vi "aotf_do_waveform_multiD.vi"(0 "Actual Sweep Time (µS)":u32, 5 "Sweep Interval (µS)":u32, 7 "Number of Slices":u32, 9 "Left Padding":u32, 11 "Right Padding":u32) -> (8 "Digital Waveform Graph":digitalwaveform(graph))   [LabVIEW 2013]
uses:
  <vilib>/Waveform/DWDTOps.llb/Digital Pattern Generator (Single Value).vi
  <vilib>/Waveform/DWDTOps.llb/DWDT Append Digital Samples.vi
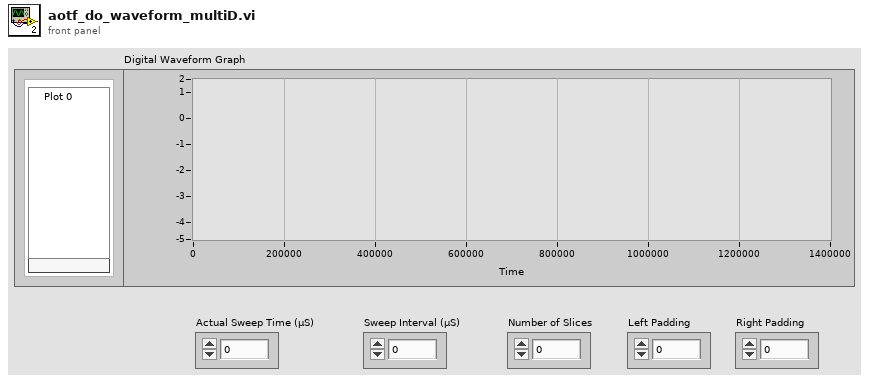
[diagram p1: front panel]
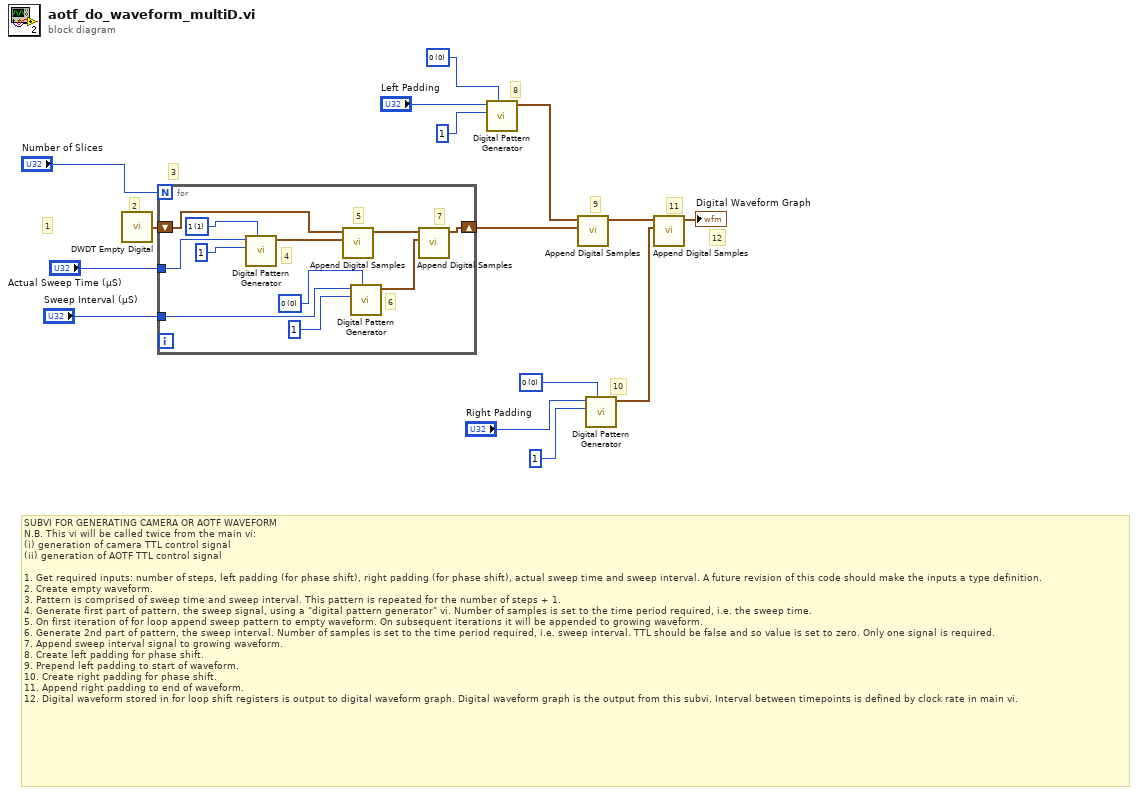
[diagram p0: block diagram]
diagram:
  w7 = u8 0 items=["0", "1", "Z", "L", "H", "X", "T", "V"] ("value")
  w10 = u8 0 items=["0", "1", "Z", "L", "H", "X", "T", "V"] ("value")
  # "12"
  # "11"
  # "10"
  # "9"
  # "8"
  # "3"
  # "2"
  # "1"
  # "SUBVI FOR GENERATING CAMERA OR AOTF WAVEFORM\nN.B. This vi will be called twice from the main vi: \n(i) generation of camera TTL control signal\n(ii) generation of AOTF TTL control signal\n\n1. Get required inputs: number of steps, left padding (for phase shift), right padding (for phase shift), actual sweep time and sweep interval. A future revision of this code should make the inputs a type definition.\n2. Create empty waveform.\n3. Pattern is comprised of sweep time and sweep interval. This pattern is repeated for the number of steps + 1.\n4. Generate first part of pattern, the sweep signal, using a \"digital pattern generator\" vi. Number of samples is set to the time period required, i.e. the sweep time.\n5. On first iteration of for loop append sweep pattern to empty waveform. On subsequent iterations it will be appended to growing waveform.\n6. Generate 2nd part of pattern, the sweep interval. Number of samples is set to the time period required, i.e. sweep interval. TTL should be false and so value is set to zero. Only one signal is required. \n7. Append sweep interval signal to growing waveform.\n8. Create left padding for phase shift.\n9. Prepend left padding to start of waveform.\n10. Create right padding for phase shift.\n11. Append right padding to end of waveform.\n12. Digital waveform stored in for loop shift registers is output to digital waveform graph. Digital waveform graph is the output from this subvi. Interval between timepoints is defined by clock rate in main vi."
  n1 = call <vilib>:"DWDT Empty Digital.vi"() -> ("digital waveform out"=w15:digitalwaveform)  [unwired: 5 in]
  n2 = for {
    N: "Number of Slices" -> [_]
    shift-right: [w16] -> w5
    shift-left: w15 -> [w17]
    tunnel: "Actual Sweep Time (µS)" -> [w20]
    tunnel: "Sweep Interval (µS)" -> [w19]
    w24 = u8 0 items=["0", "1", "Z", "L", "H", "X", "T", "V"] ("value")
    w26 = u8 1 items=["0", "1", "Z", "L", "H", "X", "T", "V"] ("value")
    # "7"
    # "6"
    # "5"
    # "4"
    n3 = call-poly <vilib>:"Digital Pattern Generator.vi"("value"=w26, "number of signals"=u32 1, "number of samples"=w20) -> ("digital waveform"=w22:digitalwaveform)  [unwired: 7 in, 1 out]
    n4 = call-poly <vilib>:"Append Digital Samples.vi"("digital waveform B"=w22, "digital waveform A"=w17) -> ("digital waveform out"=w21:digitalwaveform)  [unwired: 8 in, 1 out]
    n5 = call-poly <vilib>:"Digital Pattern Generator.vi"("value"=w24, "number of signals"=u32 1, "number of samples"=w19) -> ("digital waveform"=w18:digitalwaveform)  [unwired: 7 in, 1 out]
    n6 = call-poly <vilib>:"Append Digital Samples.vi"("digital waveform B"=w18, "digital waveform A"=w21) -> ("digital waveform out"=w16:digitalwaveform)  [unwired: 8 in, 1 out]
  }
  n7 = call-poly <vilib>:"Digital Pattern Generator.vi"("value"=w7, "number of signals"=u32 1, "number of samples"="Left Padding") -> ("digital waveform"=w6:digitalwaveform)  [unwired: 7 in, 1 out]
  n8 = call-poly <vilib>:"Append Digital Samples.vi"("digital waveform B"=w5, "digital waveform A"=w6) -> ("digital waveform out"=w4:digitalwaveform)  [unwired: 8 in, 1 out]
  n9 = call-poly <vilib>:"Digital Pattern Generator.vi"("value"=w10, "number of signals"=u32 1, "number of samples"="Right Padding") -> ("digital waveform"=w3:digitalwaveform)  [unwired: 7 in, 1 out]
  n10 = call-poly <vilib>:"Append Digital Samples.vi"("digital waveform B"=w3, "digital waveform A"=w4) -> ("digital waveform out"=→"Digital Waveform Graph":digitalwaveform)  [unwired: 8 in, 1 out]
